vi "Pump Status.vi"(8 "error in (no error)":errorcluster, 11 "VICI Settings":T1) -> (0 "error out":errorcluster, 1 "Connection Error":bool, 2 "Pump On?":enum16{"Off", "On", "Not Initialized"}(ring), 3 "VICI Settings":T1)   [LabVIEW 2018, in "VICI M6 M50 Party Mode.lvlib"]
uses:
  VICI M6 M50 Party Mode.lvlib
  Settings Cluster.ctl
  <vilib>/Instr/_visa.llb/VISA Flush IO Buffer Mask.ctl
  <vilib>/Instr/_visa.llb/VISA Configure Serial Port (Instr).vi
panel:
  out "result string":string
  out "read buffer":string
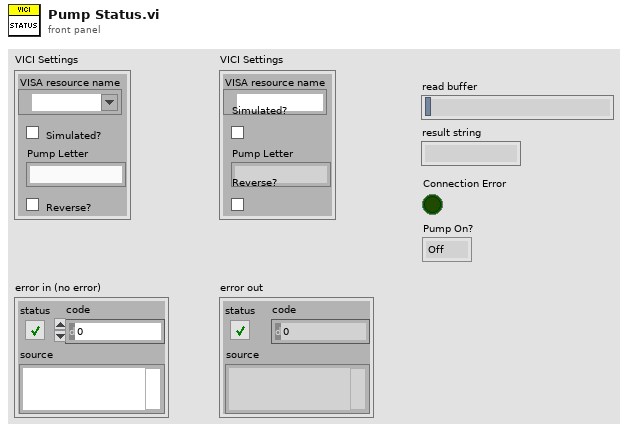
[diagram p1: front panel]
types:
  T1 = typedef "VICI M6 M50 Party Mode.lvlib/Settings Cluster.ctl" = cluster{"VISA resource name":refnum<visa-resource-name>, "Simulated?":bool, "Pump Letter":string, "Reverse?":bool}
  T2 = typedef "VISA Flush IO Buffer Mask.ctl" = u16
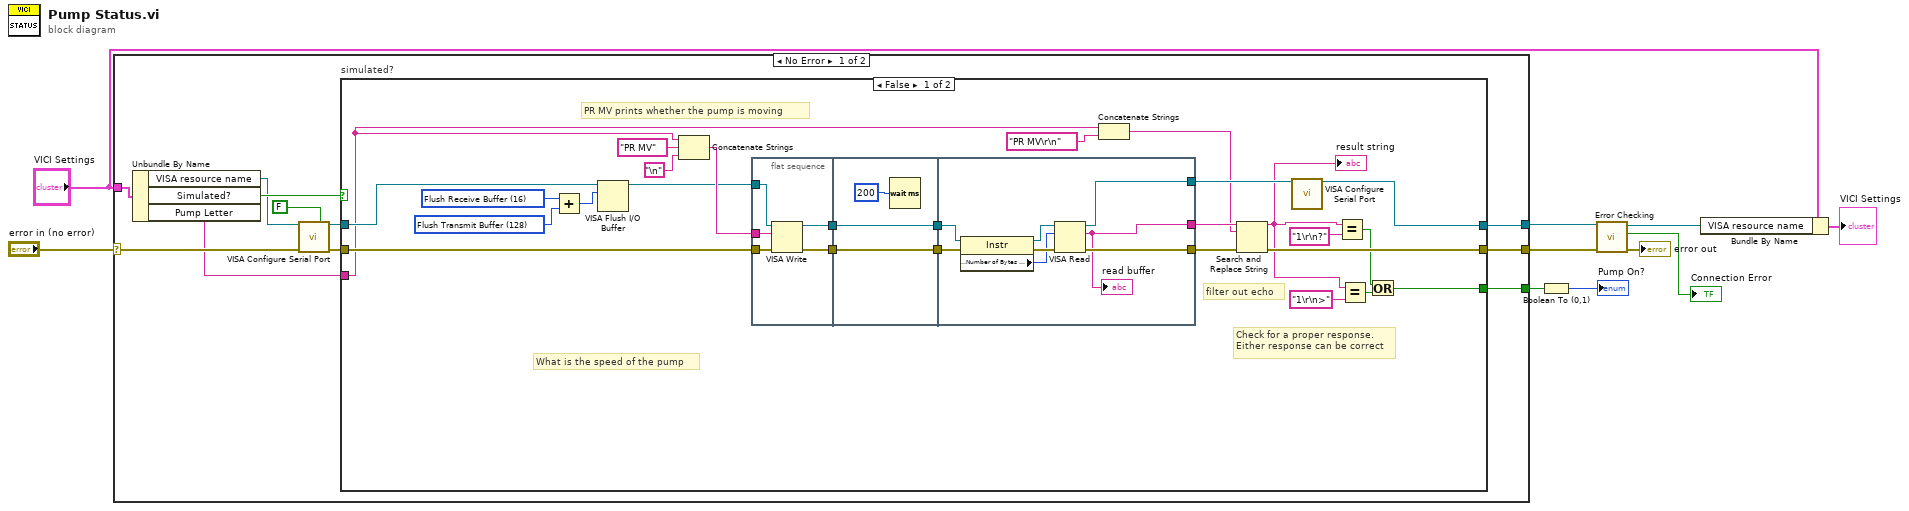
[diagram p0: block diagram]
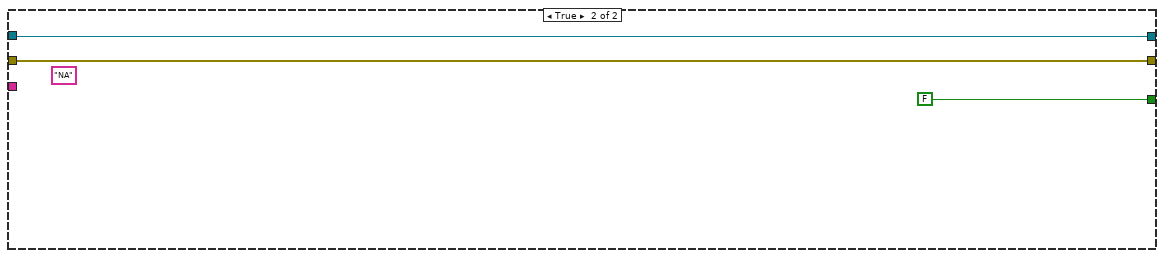
[diagram p2: hidden frame]
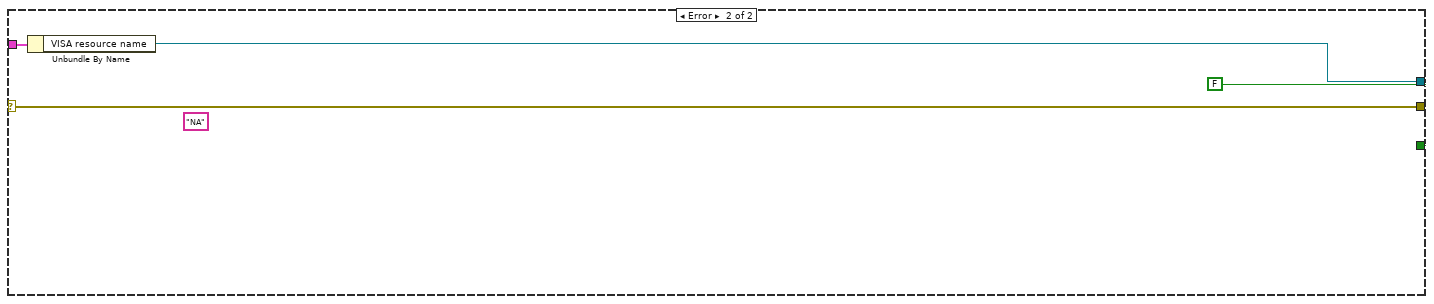
[diagram p3: hidden frame]
diagram:
  n1 = case shown="No Error" "error in (no error)" {
    selector: "error in (no error)" -> [w14 w71]
    tunnel: [w21 w71] -> w8
    tunnel: "VICI Settings" -> [w20 w70]
    tunnel: [w19 w69] -> w5
    tunnel: [w12 FALSE] -> w2
    frame No Error {
      n2 = Unbundle By Name(w20) -> ("VISA resource name"=w17:refnum<visa-resource-name>, "Simulated?"=w18:bool, "Pump Letter"=w11:string)
      n3 = call-poly "VISA Configure Serial Port"("VISA resource name"=w17, "Enable Termination\nChar (T)"=FALSE ("Enable Termination\nChar (T)"), "error in (no error)"=w14) -> ("VISA resource name out"=w16:refnum<visa-resource-name>, "error out"=w13:errorcluster)  [unwired: 11 in]
      n4 = case "simulated?" shown="False" w18 {
        tunnel: [w36 w67] -> w21
        tunnel: [w39 w65] -> w19
        tunnel: w13 -> [w24 w67]
        tunnel: w16 -> [w44 w65]
        tunnel: [w25 FALSE] -> w12
        tunnel: w11 -> [w22 _]
        frame False {
          w41 = T2 128 items=["Flush Receive Buffer"=16, "Write Transmit Buffer to Device"=32, "Flush Receive Buffer (No I/O)"=64, "Flush Transmit Buffer"=128] ("Mask")
          w42 = T2 16 items=["Flush Receive Buffer"=16, "Write Transmit Buffer to Device"=32, "Flush Receive Buffer (No I/O)"=64, "Flush Transmit Buffer"=128] ("Mask")
          # "What is the speed of the pump"
          # "filter out echo"
          # "Check for a proper response. \nEither response can be correct"
          # "PR MV prints whether the pump is moving"
          n5 = Add(x=w42, y=w41) -> (x+y=w43:T2)
          n6 = VISA Flush I/O Buffer(VISA resource name=w44, mask (16)=w43) -> (VISA resource name out=w23:refnum<visa-resource-name>)  [unwired: 1 in, 1 out]
          n7 = Concatenate Strings(w22, "PR MV" ("string"), "\n") -> (w32:string)
          n8 = flat-sequence {
            tunnel: [w51] -> w48
            tunnel: [w52] -> w47
            tunnel: [w49] -> _
            tunnel: w32 -> [w53]
            tunnel: w23 -> [w50]
            tunnel: w24 -> [w49]
            tunnel: w48 -> [w54]
            tunnel: w47 -> [w56]
            tunnel: [w56] -> w46
            tunnel: [w54] -> w45
            tunnel: w46 -> [w63]
            tunnel: w45 -> [w62]
            tunnel: [w58] -> w38
            tunnel: [w64] -> w37
            tunnel: [w57] -> w40
            frame #0 {
              n9 = VISA Write(VISA resource name=w50, write buffer=w53, error in (no error)=w49) -> (VISA resource name out=w51:refnum<visa-resource-name>, error out=w52:errorcluster)  [unwired: 1 out]
            }
            frame #1 {
              n10 = Wait (ms)(milliseconds to wait=u32 200) -> ()  [unwired: 1 out]
            }
            frame #2 {
              n11 = property class="Instr"(reference=w62, error in=w63) -> (reference out=w61:refnum<visa-resource-name>, error out=w60:errorcluster, "Serial Settings:Number of Bytes at Serial Port"=w59:u32)
              n12 = VISA Read(VISA resource name=w61, byte count=w59, error in (no error)=w60) -> (VISA resource name out=w57:refnum<visa-resource-name>, read buffer=w58:string, error out=w64:errorcluster)  [unwired: 1 out]
              "read buffer" <- w58
            }
          }
          n13 = Concatenate Strings(w22, "PR MV\r\n" ("search string")) -> (w30:string)
          n14 = Search and Replace String(input string=w38, search string=w30, error in=w37) -> (result string=w28:string, error out=w36:errorcluster)  [unwired: 5 in, 2 out]
          "result string" <- w28
          n15 = call-poly "VISA Configure Serial Port"("VISA resource name"=w40) -> ("VISA resource name out"=w39:refnum<visa-resource-name>)  [unwired: 13 in, 1 out]
          n16 = Equal?(x=w28, y="1\r\n?") -> (x = y?=w29:bool)
          n17 = Equal?(x=w28, y="1\r\n>") -> (x = y?=w27:bool)
          n18 = Or(x=w29, y=w27) -> (x .or. y?=w25:bool)
        }
        frame True {
          (unwired) "Nan" ("result string")
          (unwired) "NA" ("read buffer")
        }
      }
    }
    frame Error {
      (unwired) "Nan" ("result string")
      (unwired) "NA" ("read buffer")
      n19 = Unbundle By Name(w70) -> ("VISA resource name"=w69:refnum<visa-resource-name>)
    }
  }
  n20 = Boolean To (0,1)(Boolean=w2) -> (0, 1=→"Pump On?":i16)
  n21 = call "Error Checking.vi"("error in (no error)"=w8, "VISA resource name"=w5) -> ("error out"=→"error out":errorcluster, "Connection Error"=→"Connection Error":bool, "VISA resource name"=w4:refnum<visa-resource-name>)  [unwired: 7 in]
  n22 = Bundle By Name(cluster="VICI Settings", "VISA resource name"=w4) -> (→"VICI Settings":T1)
